vi "OpenQDInstrument.vi"(4 "Remote":bool, 5 "IP Address":string="127.0.0.1", 7 "Instrument Type":i32(ring) items=["PPMS", "VersaLab", "DynaCool", "SVSM"], 8 "error in (no error)":errorcluster) -> (2 "error out":errorcluster, 3 "Instrument Ref":refnum<k24>)   [LabVIEW 2016]
uses:
  C:/user/patrick/hg/levylab_inst_ppms2/lvsrc/PPMS/lvsrc/QDInstrument_LabView/QDInstrument.dll
  QDInstrument.dll
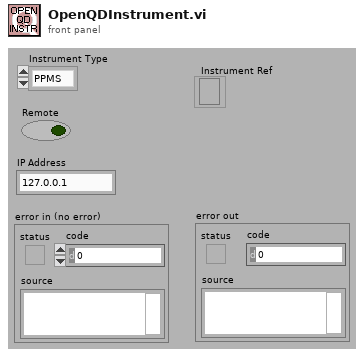
[diagram p1: front panel]
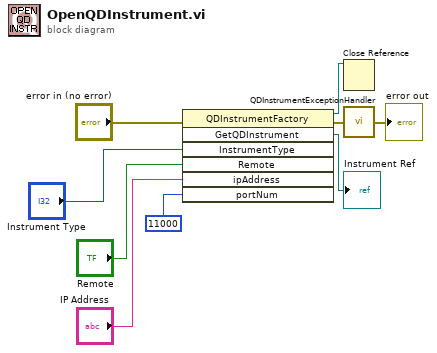
[diagram p0: block diagram]
diagram:
  n1 = invoke class="QDInstrumentFactory" method="GetQDInstrument"(error in="error in (no error)", "InstrumentType"="Instrument Type", "Remote"="Remote", "ipAddress"="IP Address", "portNum"=u16 11000 ("Port Number")) -> (reference out=w4:refnum<k24>, error out=w3:errorcluster, "GetQDInstrument"=→"Instrument Ref":refnum<k24>)  [unwired: 2 in, 4 out]
  n2 = Close Reference(reference=w4) -> ()  [unwired: 1 in, 1 out]
  n3 = call "QDInstrumentExceptionHandler.vi"("Error in"=w3) -> ("Error out"=→"error out":errorcluster)
